vi "myXi_ExtractBitArray.vi"(11 "Array":u8[](array[numeric])) -> (3 "(hi.lo) 2":u16[](array[numeric]) format="%b")   [LabVIEW 2018]
panel:
  out "Numeric":dbl[unit]
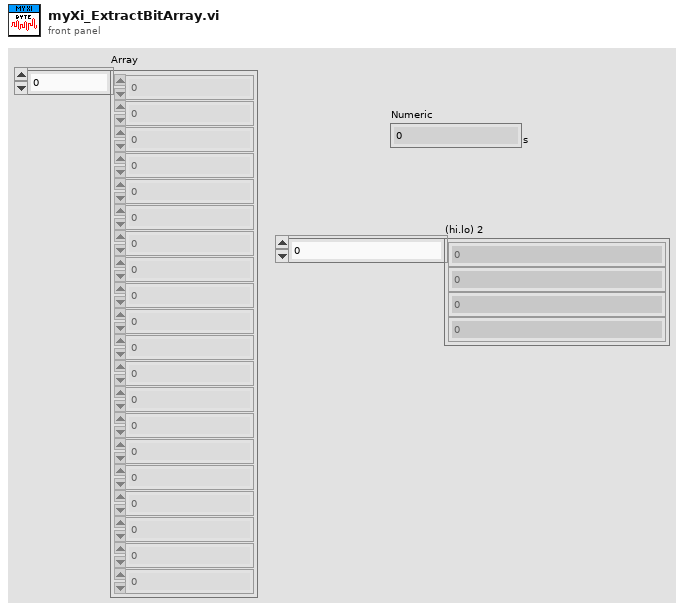
[diagram p1: front panel]
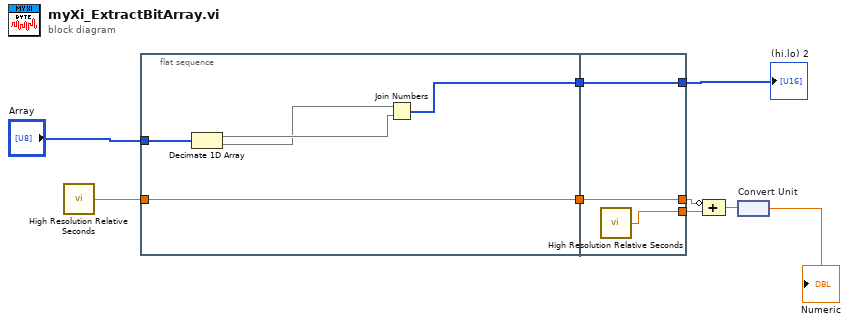
[diagram p0: block diagram]
diagram:
  n1 = call <vilib>:"High Resolution Relative Seconds.vi"() -> ("relative seconds"=w9:dbl)
  n2 = flat-sequence {
    tunnel: "Array" -> [w14]
    tunnel: w9 -> [w13]
    tunnel: [w13] -> w7
    tunnel: [w11] -> w1
    tunnel: [w17] -> w8
    tunnel: w7 -> [w16]
    tunnel: [w16] -> w6
    tunnel: [w15] -> w2
    tunnel: w1 -> [w15]
    frame #0 {
      n3 = Decimate 1D Array(w14) -> (w12:u8[], w10:u8[])
      n4 = Join Numbers(hi=w10, lo=w12) -> ((hi.lo)=w11:u16[])
    }
    frame #1 {
      n5 = call <vilib>:"High Resolution Relative Seconds.vi"() -> ("relative seconds"=w17:dbl)
    }
  }
  n6 = Compound Arithmetic op=ADD(invert w6, w8) -> (w5:dbl)
  n7 = node "Convert Unit"(w5) -> (→"Numeric":dbl[unit])
  "(hi.lo) 2" <- w2
